vi "Connect Terminals to Method VI.vi"(8 "error in (no error)":errorcluster, 11 "DVR VI Path":path=path "D:/GitHub/LabVIEW/SLL/Tools/Class DVR API Generator/Example/APIs/Sample Class Method API.vi") -> (0 "error out":errorcluster)   [LabVIEW 2016, in "SLL Class DVR API Generator.lvlib"]
uses:
  SLL Class DVR API Generator.lvlib
  <vilib>/Utility/traverseref.llb/TRef TravTarget.ctl
  <vilib>/Utility/traverseref.llb/VI Scripting - Traverse.lvlib
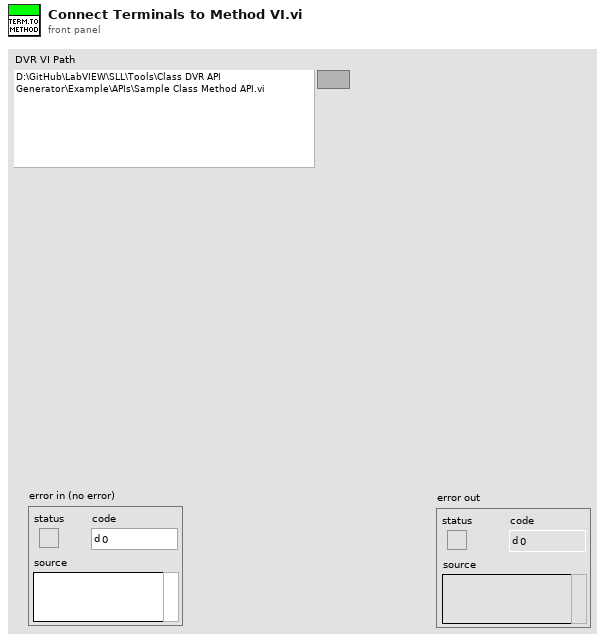
[diagram p1: front panel]
types:
  T1 = typedef "TRef TravTarget.ctl" = enum16{"FP", "BD", "Other"}
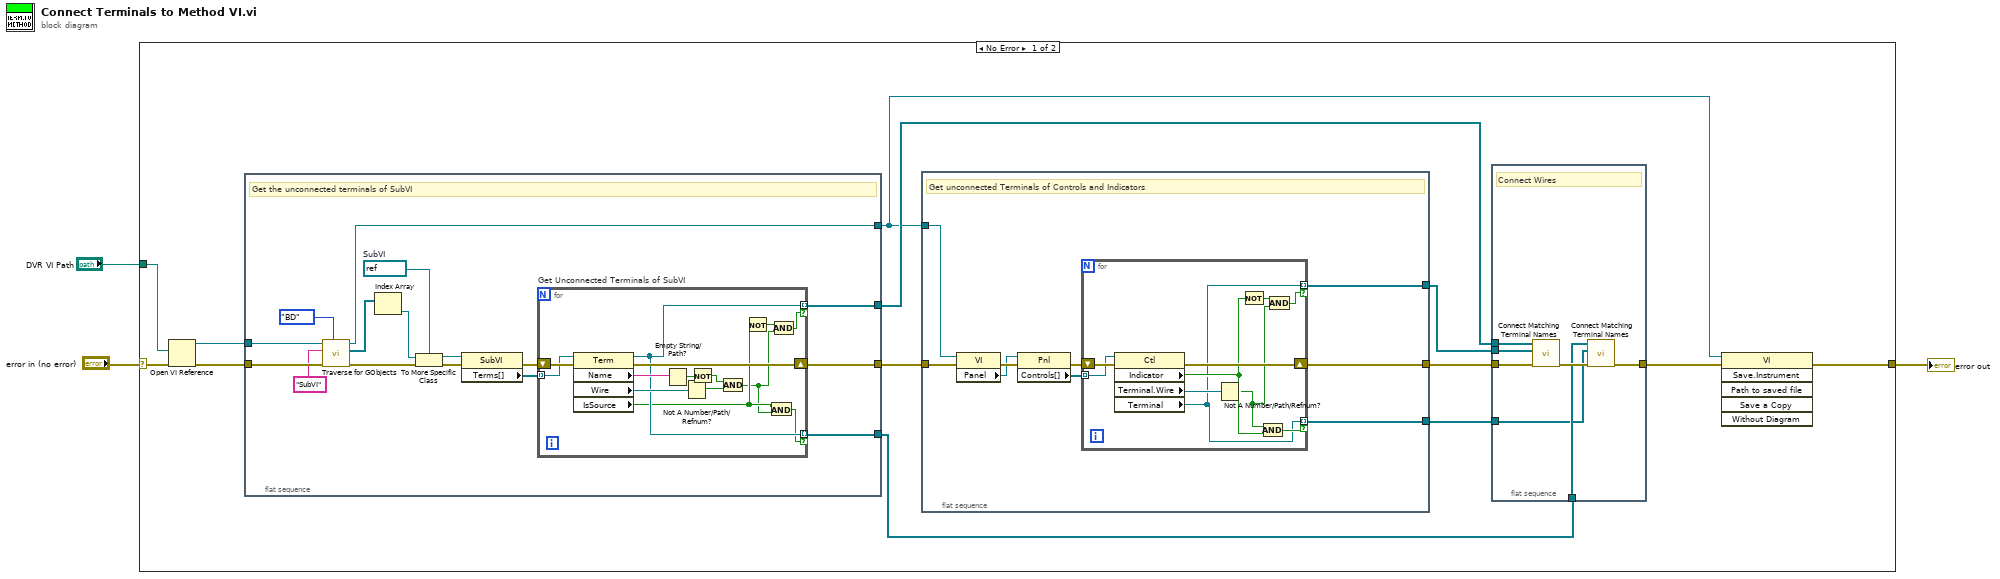
[diagram p0: block diagram]
diagram:
  n1 = case shown="No Error" "error in (no error)" {
    selector: "error in (no error)" -> [w16 w73]
    tunnel: [w5 w73] -> w2
    tunnel: "DVR VI Path" -> [w14 _]
    frame No Error {
      n2 = Open VI Reference(vi path=w14, error in (no error)=w16) -> (vi reference=w13:refnum<vi>, error out=w15:errorcluster)  [unwired: 4 in]
      n3 = flat-sequence {
        tunnel: w15 -> [w58]
        tunnel: w13 -> [w55]
        tunnel: [w47] -> w12
        tunnel: [w45] -> w9
        tunnel: [w44] -> w7
        tunnel: [w43] -> w4
        frame #0 {
          w50 = refnum<vi> refnum  # SubVI
          # "Get the unconnected terminals of SubVI"
          n4 = call <vilib>:"Traverse for GObjects.vi"("Traverse Target"=TRef_TravTarget."BD", "error in (no error)"=w58, "Class Name"="SubVI" ("name/order"), "VI Refnum"=w55) -> ("error out"=w57:errorcluster, "References"=w53:refnum<vi>[], "dup VI Refnum"=w43:refnum<vi>)  [unwired: 4 in, 1 out]
          n5 = Index Array(array=w53) -> (element=w51:refnum<vi>)  [unwired: 1 in]
          n6 = To More Specific Class(target class=w50, reference=w51, error in=w57) -> (specific class reference=w48:refnum<vi>, error out=w52:errorcluster)
          n7 = property class="SubVI"(reference=w48, error in=w52) -> (error out=w49:errorcluster, "Terms[]"=w46:refnum<vi>[])  [unwired: 1 out]
          n8 = for "Get Unconnected Terminals of SubVI" {
            shift-right: [w71] -> w47
            shift-left: w49 -> [w72]
            tunnel: w46 -> [w70] mode=indexing
            tunnel: [w62] -> w45 mode=indexing if=w63
            tunnel: [w62] -> w44 mode=indexing if=w59
            n9 = property class="Term"(reference=w70, error in=w72) -> (reference out=w62:refnum<vi>, error out=w71:errorcluster, "Name"=w68:string, "Wire"=w69:refnum<vi>, "IsSource"=w61:bool)
            n10 = Empty String/Path?(string/path=w68) -> (empty?=w67:bool)
            n11 = Not A Number/Path/Refnum?(number/path/refnum=w69) -> (NaN/Path/Refnum?=w65:bool)
            n12 = Not(x=w67) -> (.not. x?=w66:bool)
            n13 = And(x=w66, y=w65) -> (x .and. y?=w60:bool)
            n14 = Not(x=w61) -> (.not. x?=w64:bool)
            n15 = And(x=w61, y=w60) -> (x .and. y?=w59:bool)
            n16 = And(x=w64, y=w60) -> (x .and. y?=w63:bool)
          }
        }
      }
      n17 = flat-sequence {
        tunnel: w12 -> [w32]
        tunnel: [w27] -> w11
        tunnel: w4 -> [w30]
        tunnel: [w25] -> w8
        tunnel: [w24] -> w6
        frame #0 {
          # "Get unconnected Terminals of Controls and Indicators"
          n18 = property class="VI"(reference=w30, error in=w32) -> (error out=w31:errorcluster, "Panel"=w28:refnum<vi>)  [unwired: 1 out]
          n19 = property class="Pnl"(reference=w28, error in=w31) -> (error out=w29:errorcluster, "Controls[]"=w26:refnum<vi>[])  [unwired: 1 out]
          n20 = for {
            shift-right: [w41] -> w27
            shift-left: w29 -> [w42]
            tunnel: w26 -> [w40] mode=indexing
            tunnel: [w33] -> w25 mode=indexing if=w37
            tunnel: [w33] -> w24 mode=indexing if=w36
            n21 = property class="Ctl"(reference=w40, error in=w42) -> (error out=w41:errorcluster, "Indicator"=w35:bool, "Terminal.Wire"=w39:refnum<vi>, "Terminal"=w33:refnum<vi>)  [unwired: 1 out]
            n22 = Not A Number/Path/Refnum?(number/path/refnum=w39) -> (NaN/Path/Refnum?=w34:bool)
            n23 = Not(x=w35) -> (.not. x?=w38:bool)
            n24 = And(x=w34, y=w35) -> (x .and. y?=w36:bool)
            n25 = And(x=w38, y=w34) -> (x .and. y?=w37:bool)
          }
        }
      }
      n26 = flat-sequence {
        tunnel: w11 -> [w23]
        tunnel: [w17] -> w10
        tunnel: w9 -> [w22]
        tunnel: w8 -> [w21]
        tunnel: w7 -> [w19]
        tunnel: w6 -> [w18]
        frame #0 {
          # "Connect Wires"
          n27 = call "Connect Matching Terminal Names.vi"("error in (no error)"=w23, "Terminal Set #2"=w21, "Terminal Set #1"=w22) -> ("error out"=w20:errorcluster)  [unwired: 8 in]
          n28 = call "Connect Matching Terminal Names.vi"("error in (no error)"=w20, "Terminal Set #2"=w18, "Terminal Set #1"=w19) -> ("error out"=w17:errorcluster)  [unwired: 8 in]
        }
      }
      n29 = invoke class="VI" method="Save.Instrument"(reference=w4, error in=w10) -> (error out=w5:errorcluster)  [unwired: 4 in, 5 out]
    }
    frame Error {
    }
  }
  "error out" <- w2
